vi "Value To String.vi"(8 "error in (no error)":errorcluster, 11 "NT Scalar (Numeric) in":refnum<class "NT Scalar (Numeric).lvclass">) -> (0 "error out":errorcluster, 2 "string":string, 3 "NT Scalar (Numeric) out":refnum<class "NT Scalar (Numeric).lvclass">)   [LabVIEW 2020, in "PV Access.lvlib" / "PV Data.lvlib" / "NT Scalar (Numeric).lvclass"]
uses:
  NT Scalar (Numeric).lvclass
  C:/Users/eyw68381/source/repos/pvaccess-labview/labview/source/PV Data/NT Base/NT Base.lvclass
  NT Scalar/NT Scalar.lvclass
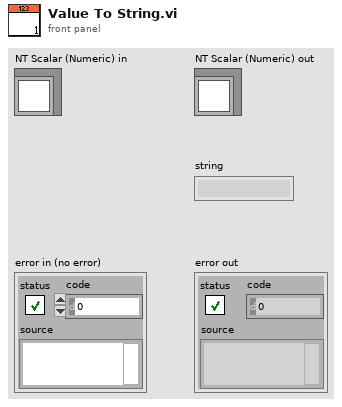
[diagram p1: front panel]
types:
  T1 = typedef "PV Access.lvlib/PV Data.lvlib/Type Code.ctl" = enum8{"Null", "Bool", "BoolA", "Int8", "Int8A", "Int16", "Int16A", "Int32", "Int32A", "Int64", "Int64A", "UInt8", "UInt8A", "UInt16", "UInt16A", "UInt32", "UInt32A", "UInt64", "UInt64A", "Float32", "Float32A", "Float64", "Float64A", "String", "StringA", "Struct", "StructA", "Union", "UnionA", "Any", "AnyA"}
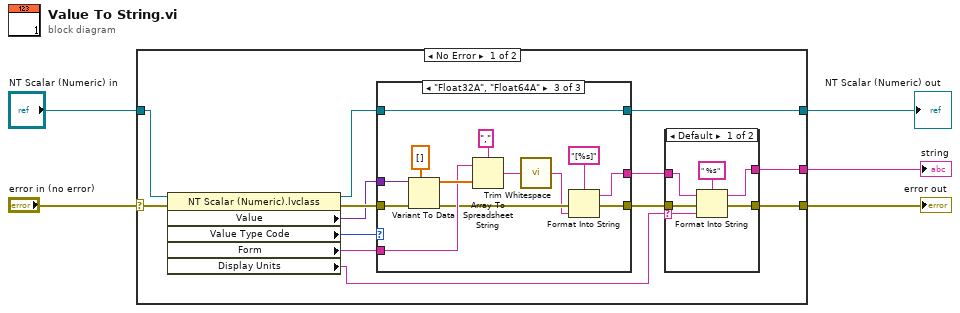
[diagram p0: block diagram]
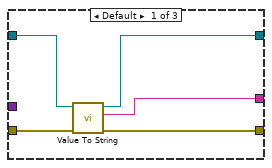
[diagram p3: hidden frame]
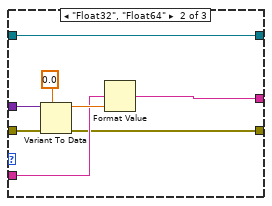
[diagram p4: hidden frame]
diagram:
  n1 = case shown="No Error" "error in (no error)" {
    selector: "error in (no error)" -> [w15 w54]
    tunnel: [w6 w54] -> w2
    tunnel: [w11 w53] -> w1
    tunnel: "NT Scalar (Numeric) in" -> [w14 w53]
    tunnel: [w9 _] -> w3
    frame No Error {
      n2 = property class="NT Scalar (Numeric).lvclass"(reference=w14, error in=w15) -> (reference out=w12:refnum<class "NT Scalar (Numeric).lvclass">, error out=w18:errorcluster, "Value"=w16:variant, "Value Type Code"=w17:T1, "Form"=w13:string, "Display Units"=w10:string)
      n3 = case shown="\"Float32A\", \"Float64A\"" w17 {
        tunnel: w18 -> [w31 w37 w51]
        tunnel: w16 -> [_ w38 w52]
        tunnel: [w28 w32 w45] -> w7
        tunnel: [w27 w33 w43] -> w8
        tunnel: w13 -> [_ w34 w48]
        tunnel: w12 -> [w30 w36 w47]
        tunnel: [w29 w36 w47] -> w11
        frame Default {
          n4 = call-parent "Value To String.vi"("error in (no error)"=w31, "NT Base in"=w30) -> ("error out"=w28:errorcluster, "string"=w27:string, "NT Base out"=w29:refnum<class "NT Scalar (Numeric).lvclass">)  [unwired: 7 in]
        }
        frame "Float32", "Float64" {
          n5 = Variant To Data(error in=w37, type=0.0, Variant=w38) -> (data=w35:dbl, error out=w32:errorcluster)
          n6 = Format Value(format string=w34, value (0)=w35) -> (output string=w33:string)  [unwired: 1 in]
        }
        frame "Float32A", "Float64A" {
          n7 = Variant To Data(error in=w51, type=dbl[] [], Variant=w52) -> (data=w49:dbl[], error out=w44:errorcluster)
          n8 = Array To Spreadsheet String(delimiter (Tab)=",", array=w49, 3:w48) -> (spreadsheet string=w41:string)
          n9 = call <vilib>:"Trim Whitespace.vi"("string"=w41) -> ("trimmed string"=w40:string)  [unwired: 1 in]
          n10 = Format Into String(format string="[%s]", error in=w44, w40) -> (resulting string=w43:string, error out=w45:errorcluster)  [unwired: 1 in]
        }
      }
      n11 = case shown="Default" w10 {
        selector: w10 -> [w20 _]
        tunnel: w8 -> [w21 w26]
        tunnel: [w19 w26] -> w9
        tunnel: w7 -> [w23 w25]
        tunnel: [w22 w25] -> w6
        frame Default {
          n12 = Format Into String(format string=" %s", initial string=w21, error in=w23, w20) -> (resulting string=w19:string, error out=w22:errorcluster)
        }
        frame "" {
        }
      }
    }
    frame Error {
    }
  }
  "error out" <- w2
  "NT Scalar (Numeric) out" <- w1
  "string" <- w3
